vi "RstCount.vi"(11 "Reset counter":bool) -> ()   [LabVIEW 2020]
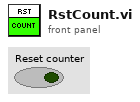
[diagram p1: front panel]
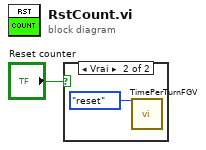
[diagram p0: block diagram]
diagram:
  n1 = case shown="Vrai" "Reset counter" {
    frame False {
    }
    frame True {
      n2 = call "TimePerTurnFGV.vi"("Énum"=enum16{"reset", "read", "home"}."reset") -> ()  [unwired: 9 in, 2 out]
    }
  }
